vi "Get Item Reference By Name.vi"(8 "error in (no error)":errorcluster, 10 "Item Name":string, 11 "Section Reference in":u64 format="%.0x") -> (0 "error out":errorcluster, 2 "Item Reference":u64 format="%.0x", 3 "Section Reference out":u64 format="%.0x", 4 "found":bool)   [LabVIEW 2013, in "Hierarchy Framework.lvlib" / "Section.lvclass"]
doc: "Searches for <B>Item Name</B> in the section specified by <B>Section Reference in</B> and, if found, returns a reference to the item."
uses:
  Section.lvclass
  Generic/Generic.lvclass
  Item/Item.lvclass
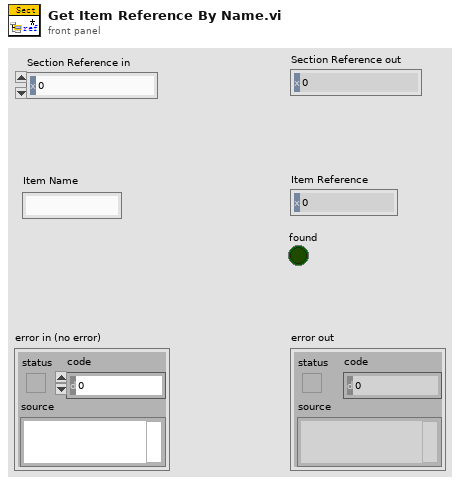
[diagram p1: front panel]
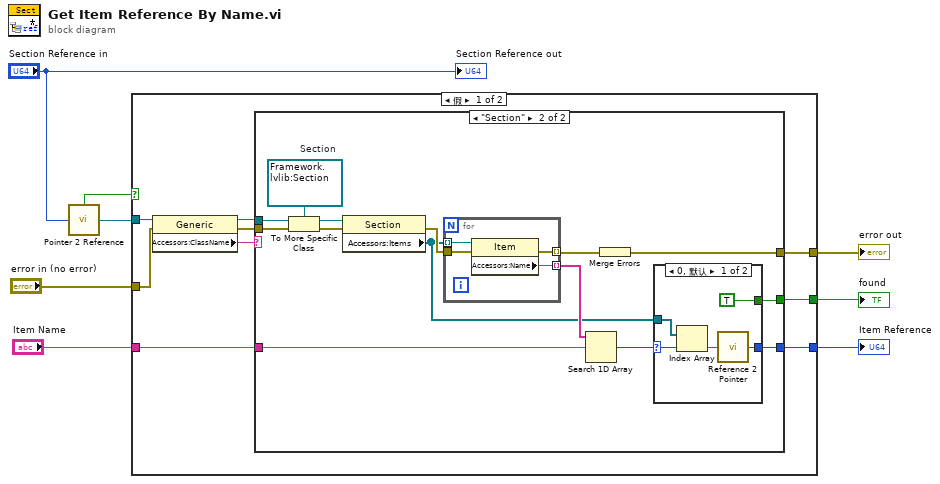
[diagram p0: block diagram]
diagram:
  n1 = call "Pointer 2 Reference.vi"("Pointer"="Section Reference in") -> ("Not A Refnum?"=w5:bool, "Generic Reference"=w4:refnum<data-value>)
  n2 = case shown="假" w5 {
    tunnel: w4 -> [w16 _]
    tunnel: "error in (no error)" -> [w15 w42]
    tunnel: [w17 w42] -> w7
    tunnel: [w11 _] -> w1
    tunnel: [w10 _] -> w3
    tunnel: "Item Name" -> [w9 _]
    frame False {
      n3 = property class="Generic"(reference=w16, error in=w15) -> (reference out=w13:refnum<data-value>, error out=w14:errorcluster, "Accessors:ClassName"=w12:string)
      n4 = case shown="\"Section\"" w12 {
        tunnel: [w18 w25] -> w17
        tunnel: w14 -> [w18 w29]
        tunnel: w13 -> [_ w28]
        tunnel: [_ w20] -> w11
        tunnel: [_ w19] -> w10
        tunnel: w9 -> [_ w23]
        frame Default {
        }
        frame "Section" {
          w32 = refnum<data-value> refnum  # Section
          n5 = To More Specific Class(target class=w32, reference=w28, error in=w29) -> (specific class reference=w31:refnum<data-value>, error out=w30:errorcluster)
          n6 = property class="Section"(reference=w31, error in=w30) -> (error out=w26:errorcluster, "Accessors:Items"=w21:refnum<data-value>[])  [unwired: 1 out]
          n7 = for {
            tunnel: w21 -> [w41] mode=indexing
            tunnel: [w40] -> w24 mode=indexing
            tunnel: w26 -> [w39]
            tunnel: [w38] -> w27 mode=indexing
            n8 = property class="Item"(reference=w41, error in=w39) -> (error out=w38:errorcluster, "Accessors:Name"=w40:string)  [unwired: 1 out]
          }
          n9 = Search 1D Array(1D array=w24, element=w23) -> (index of element=w22:i32)  [unwired: 1 in]
          n10 = Merge Errors(w27) -> (w25:errorcluster)
          n11 = case shown="0, 默认" w22 {
            selector: w22 -> [w37 _]
            tunnel: w21 -> [w36 _]
            tunnel: [w34 _] -> w20
            tunnel: [TRUE _] -> w19
            frame 0, Default {
              n12 = Index Array(array=w36, index=w37) -> (element=w35:refnum<data-value>)
              n13 = call "Reference 2 Pointer.vi"("Generic Reference"=w35) -> ("Pointer"=w34:u64)  [unwired: 1 out]
            }
            frame -1 {
            }
          }
        }
      }
    }
    frame True {
    }
  }
  "error out" <- w7
  "found" <- w3
  "Item Reference" <- w1
  "Section Reference out" <- "Section Reference in"
